vi "CSM - Fix JKISM Editor RCM Entry.vi"() -> ()   [LabVIEW 2017]
doc: "### CSM - Fix JKISM Editor RCM Entry.vi\n\nFix JKISM State Editor of Right Click Menu Entry for CSM."
panel:
  out "String":string
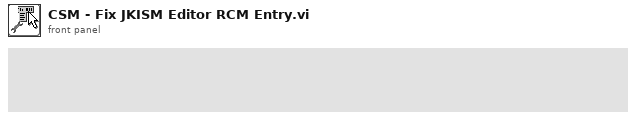
[diagram p1: front panel]
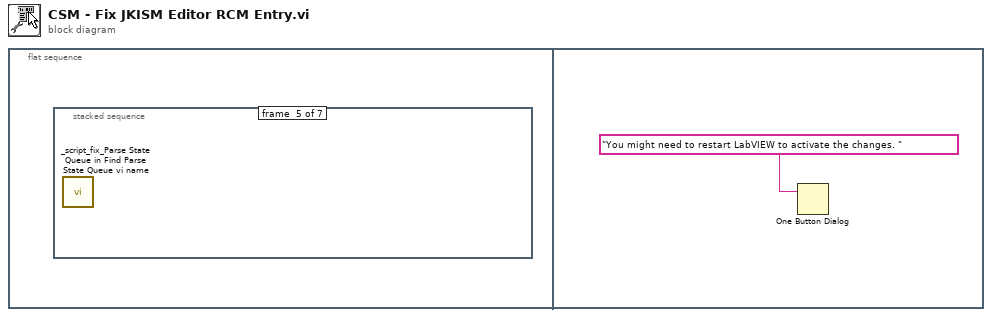
[diagram p0: block diagram]
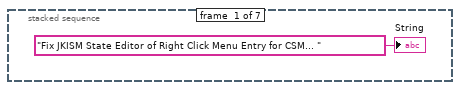
[diagram p2: hidden frame]
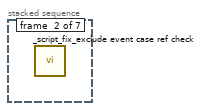
[diagram p3: hidden frame]
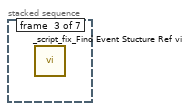
[diagram p4: hidden frame]
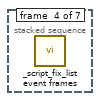
[diagram p5: hidden frame]
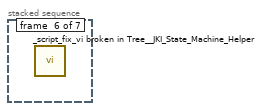
[diagram p6: hidden frame]
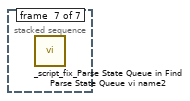
[diagram p7: hidden frame]
diagram:
  n1 = flat-sequence {
    frame #0 {
      n2 = stacked-sequence {
        frame #0 {
          "String" <- "Fix JKISM State Editor of Right Click Menu Entry for CSM... " ("String")
        }
        frame #1 {
          n3 = call "_script_fix_exclude event case ref check.vi"() -> ()  [unwired: 12 in]
        }
        frame #2 {
          n4 = call "_script_fix_Find Event Stucture Ref vi.vi"() -> ()  [unwired: 12 in]
        }
        frame #3 {
          n5 = call "_script_fix_list event frames.vi"() -> ()  [unwired: 12 in]
        }
        frame #4 {
          n6 = call "_script_fix_Parse State Queue in Find Parse State Queue vi name.vi"() -> ()  [unwired: 12 in]
        }
        frame #5 {
          n7 = call "_script_fix_vi broken in Tree__JKI_State_Machine_Helper.vi"() -> ()  [unwired: 12 in]
        }
        frame #6 {
          n8 = call "_script_fix_Parse State Queue in Find Parse State Queue vi name2.vi"() -> ()  [unwired: 12 in]
        }
      }
    }
    frame #1 {
      n9 = One Button Dialog(message="You might need to restart LabVIEW to activate the changes. ") -> ()  [unwired: 1 in, 1 out]
    }
  }
